vi "Edit Support lvproj PPL Names.vi"(8 "error in":errorcluster, 11 "custom device path":path) -> (0 "error out":errorcluster, 3 "custom device path out":path)   [LabVIEW 2020, in "Template Tool.lvlib"]
uses:
  Template Tool.lvlib
  Template Tool Global.vi
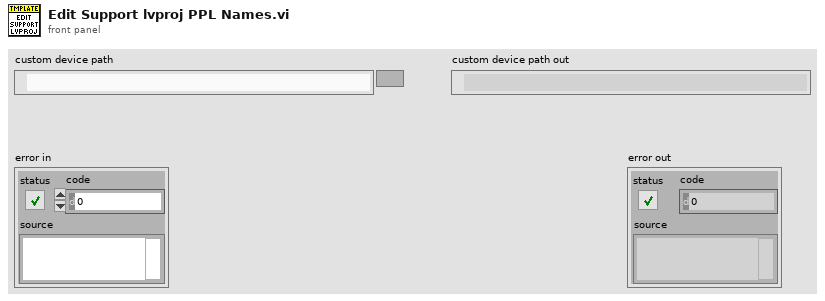
[diagram p1: front panel]
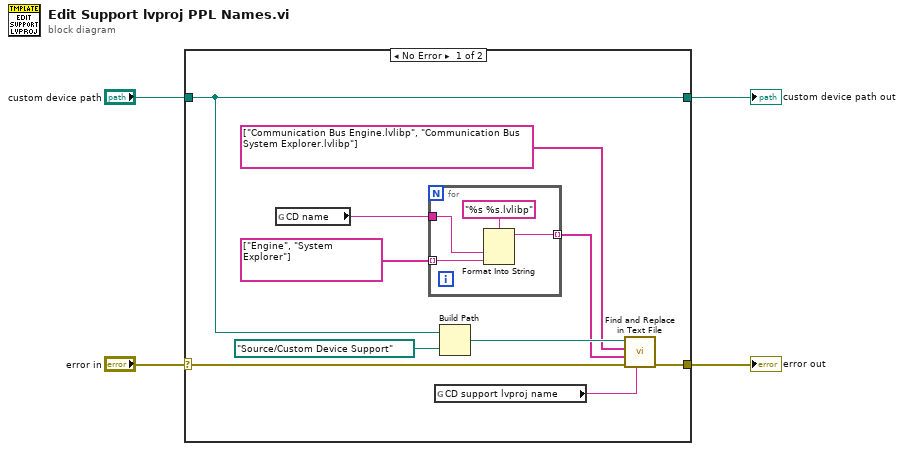
[diagram p0: block diagram]
diagram:
  n1 = case shown="No Error" "error in" {
    selector: "error in" -> [w12 w19]
    tunnel: "custom device path" -> [w13 w20]
    tunnel: [w11 w19] -> w4
    tunnel: [w13 w20] -> w1
    frame No Error {
      n2 = global read "Template Tool Global.vi" "CD name"() -> (w6:string)
      n3 = for {
        tunnel: string[] ["Engine", "System Explorer"] -> [w17] mode=indexing
        tunnel: w6 -> [w16]
        tunnel: [w15] -> w5 mode=indexing
        n4 = Format Into String(format string="%s %s.lvlibp" ("string"), w16, w17) -> (resulting string=w15:string)  [unwired: 2 in, 1 out]
      }
      n5 = global read "Template Tool Global.vi" "CD support lvproj name"() -> (w8:string)
      n6 = Build Path(base path=w13, name or relative path=path "Source/Custom Device Support") -> (appended path=w10:path)
      n7 = call "Find and Replace in Text File.vi"("file name"=w8, "error in"=w12, "replace array"=w5, "find array"=string[] ["Communication Bus Engine.lvlibp", "Communication Bus System Explorer.lvlibp"], "folder path"=w10) -> ("error out"=w11:errorcluster)  [unwired: 5 in, 1 out]
    }
    frame Error {
    }
  }
  "error out" <- w4
  "custom device path out" <- w1
